vi "Dequeue Message.vi"(8 "error in (no error)":errorcluster, 9 "timeout in ms (-1)":i32=-1, 11 "Queue in":refnum<queue>) -> (0 "error out":errorcluster, 1 "Message Data":variant, 2 "Message":string, 3 "Queue out":refnum<queue>)   [LabVIEW 2020, in "Debugger.lvclass"]
uses:
  Debugger.lvclass
  Debugger.lvclass/Debugger.ctl
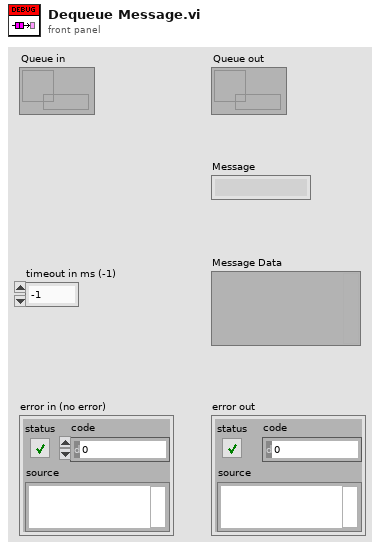
[diagram p1: front panel]
types:
  T1 = cluster{"Message":string, "Message Data":variant}
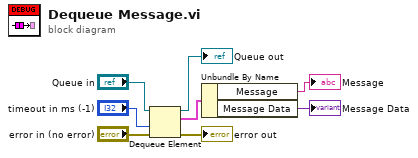
[diagram p0: block diagram]
diagram:
  n1 = Dequeue Element(queue="Queue in", timeout in ms (-1)="timeout in ms (-1)", error in (no error)="error in (no error)") -> (queue out=→"Queue out":refnum<queue>, element=w2:T1, error out=→"error out":errorcluster)  [unwired: 1 out]
  n2 = Unbundle By Name(w2) -> ("Message"=→"Message":string, "Message Data"=→"Message Data":variant)
